vi "辗转相除改进版？？.vi"() -> ()   [LabVIEW 2017]
panel:
  out "GCD":i32
  in  "n":i32
  in  "m":i32
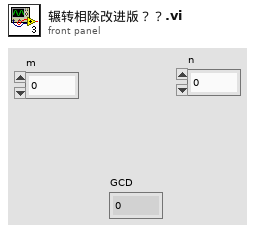
[diagram p1: front panel]
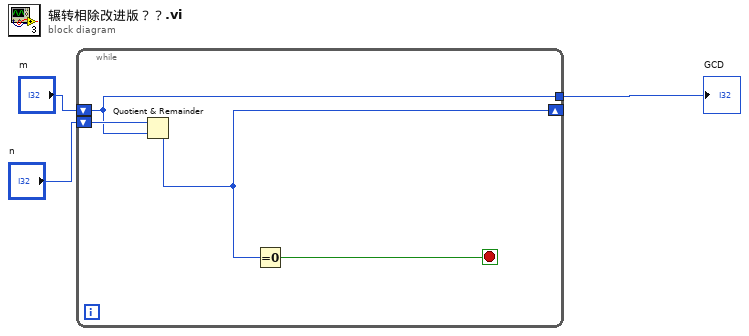
[diagram p0: block diagram]
diagram:
  n1 = while {
    shift-right: [w6] -> _
    shift-left: "m" -> [w4]
    shift-left: "n" -> [w5]
    tunnel: [w4] -> w1
    stop <- w7 stop-if-true
    n2 = Quotient & Remainder(x=w5, y=w4) -> (x-y*floor(x/y)=w6:i32)  [unwired: 1 out]
    n3 = Equal To 0?(x=w6) -> (x = 0?=w7:bool)
  }
  "GCD" <- w1
